vi "RadarAudioPlug+bluetooth.vi"() -> ()   [LabVIEW 2012]
doc: "This VI illustrates how to acquire sound samples continuously from a specified device. It requires the use of a microphone attached to the sound card. You can specify the number of samples to acquire, sample rate, number of channels and a bit rate per sample. The VI also plots the raw data as the acquisition is made."
uses:
  <vilib>/sound2/lvsound2.llb/Sound Data Format.ctl
  <vilib>/Analysis/4window.llb/windowTd.ctl
  <vilib>/sound2/lvsound2.llb/Sampling Mode.ctl
  <vilib>/Instr/_visa.llb/VISA Configure Serial Port (Instr).vi
  <vilib>/sound2/lvsound2.llb/Sound Input Read (DBL).vi
  <vilib>/gmath/NI_Gmath.lvlib
  <vilib>/ptbypt/NI_PtbyPt.lvlib
  <vilib>/Analysis/NI_AALPro.lvlib
panel:
  in  "Enable Termination\nChar (T)":bool=TRUE
  out "read buffer":string
  out "I/Q signal":dynamicdata(graph)
  in  "?":bool
  in  "flow control":u16(ring) items=["None"=0, "XON/XOFF"=1, "RTS/CTS"=2, "DTR/DSR"=4]
  in  "Input\nbuffer size":u32=4096
  in  "termination char\n(0xA = '\\n' = LF)":u8=10 format="%.0x"
  in  "timeout (ms)":u32=10000
  in  "stop bits":u16(ring)=10 items=["1.0"=10, "1.5"=15, "2.0"=20]
  in  "parity":u16(ring) items=["None", "Odd", "Even", "Mark", "Space"]
  in  "data bits":u16=8 min=5 max=8 step=1
  in  "VISA resource name":refnum<visa-resource-name>="COM1"
  in  "baud rate":u32=115200
  in  "start time":timestamp
  in  "stop time":timestamp
  out "STFT Spectrogram":dbl[][](graph)
  in  "Save data":bool=TRUE caption="Enable"
  in  "window info":cluster{"type":T1, "length":i32}={"type"=1, "length"=64} {"type" items=["Rectangle"=0, "Hanning"=1, "Hamming"=2, "Blackman-Harris"=3, "Exact Blackman"=4, "Blackman"=5, "Flat Top"=6, "4 Term B-Harris "=7, "7 Term B-Harris"=8, "Low Sidelobe"=9, "Blackman Nuttall"=11, "Triangle"=30, "Bartlett-Hanning"=31, "Bohman"=32, "Parzen"=33, "Welch"=34, "Kaiser"=60, "Dolph-Chebyshev"=61, "Gaussian"=62]}
  in  "time-freq sampling info":cluster{"time steps":i32, "frequency bins":i32}={"time steps"=-1, "frequency bins"=512}
  in  "Sound Format":T2={"sample rate (S/s)"=22050.0, "number of channels"=2, "bits per sample"=16}
  out "Raw Data":waveform(dbl)[](graph)
  in  "stop":bool
  in  "Device ID":u32 format="%.0x"
  in  "Number of Samples/ch":i32=5000
  # "Configuration"
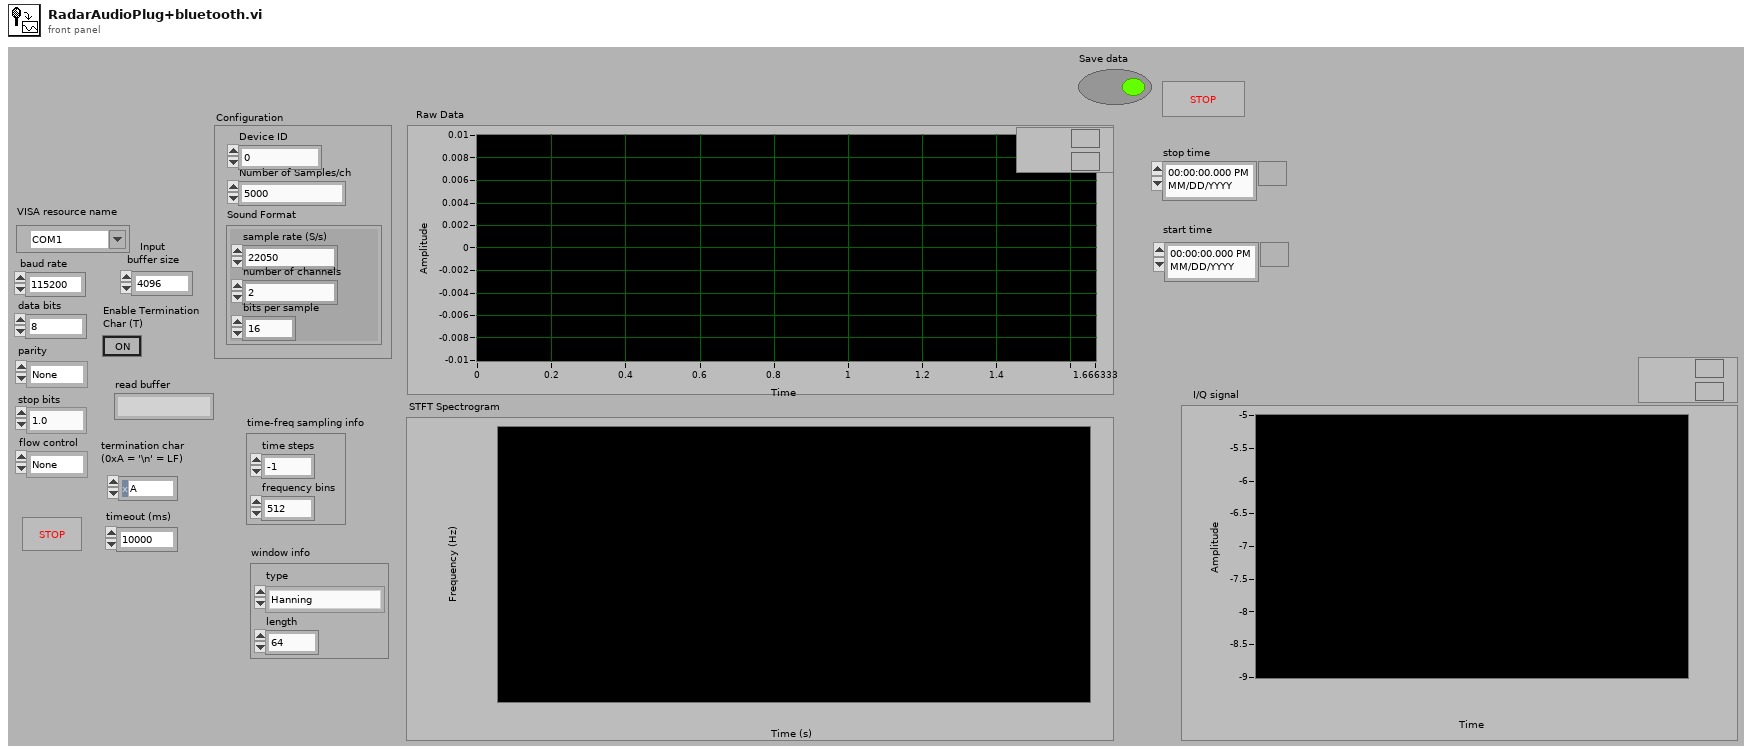
[diagram p1: front panel]
types:
  T1 = typedef "NI_AALPro.lvlib/windowTd.ctl" = u32
  T2 = typedef "Sound Data Format.ctl" = cluster{"sample rate (S/s)":dbl, "number of channels":i32, "bits per sample":i32}
  T3 = typedef "Sampling Mode.ctl" = i32
  T4 = typedef "Sound Input Task ID.ctl" = u32
  T5 = enum16{"fire", "rainbow", "grey", "inverse grey", "ice", "original"}
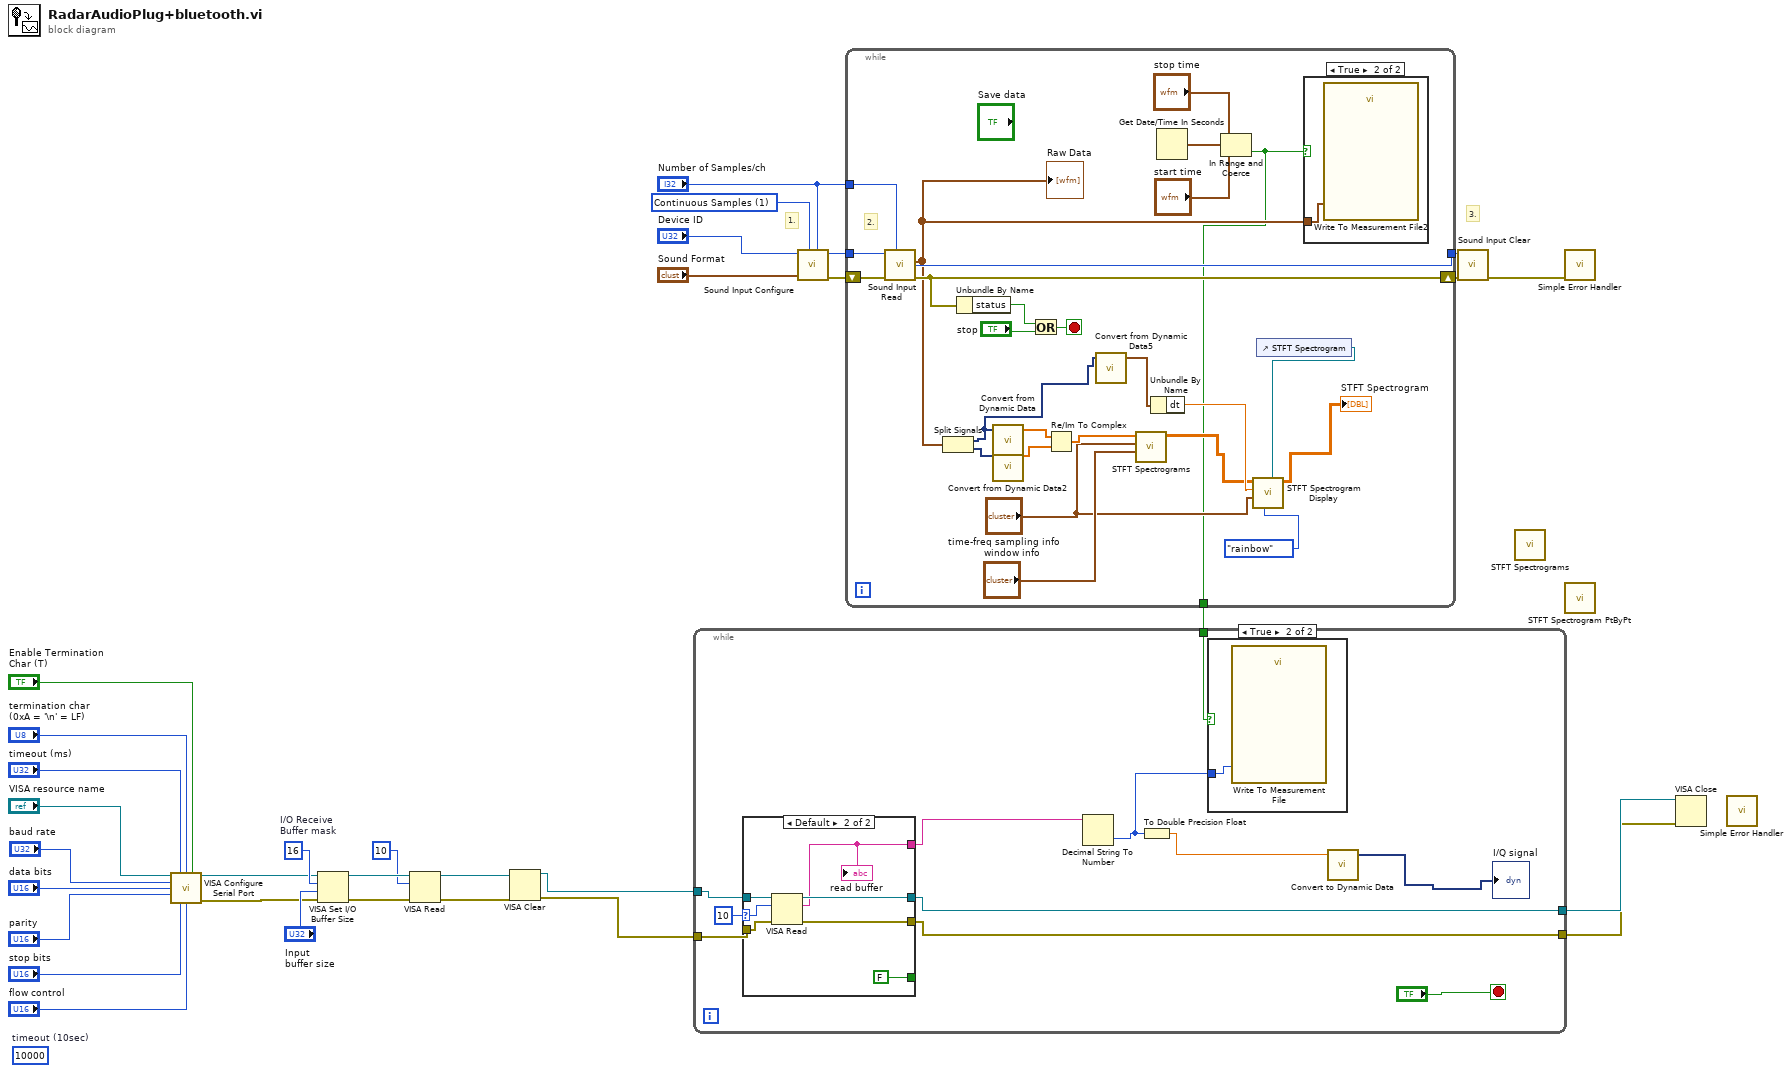
[diagram p0: block diagram]
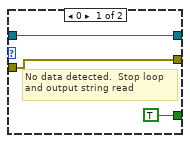
[diagram p3: hidden frame]
diagram:
  (unwired) u32 10000  # timeout (10sec)
  w18 = u16 16  # I/O Receive Buffer mask
  w27 = T3 1 items=["Finite Samples", "Continuous Samples"] ("sample mode")
  # "3."
  # "1."
  n1 = call-poly "VISA Configure Serial Port"("VISA resource name"="VISA resource name", "timeout (10sec)"="timeout (ms)", "termination char\n(0xA = '\\n' = LF)"="termination char\n(0xA = '\\n' = LF)", "Enable Termination\nChar (T)"="Enable Termination\nChar (T)", "baud rate (9600)"="baud rate", "data bits (8)"="data bits", "parity (0:none)"="parity", "stop bits (10: 1 bit)"="stop bits", "flow control (0:none)"="flow control") -> ("VISA resource name out"=w13:refnum<visa-resource-name>, "error out"=w12:errorcluster)  [unwired: 1 in, 4 out]
  n2 = VISA Set I/O Buffer Size(VISA resource name=w13, mask (16)=w18, size (4096)="Input\nbuffer size", error in (no error)=w12) -> (VISA resource name out=w11:refnum<visa-resource-name>, error out=w10:errorcluster)
  n3 = VISA Read(VISA resource name=w11, byte count=u32 10, error in (no error)=w10) -> (VISA resource name out=w7:refnum<visa-resource-name>, error out=w6:errorcluster)  [unwired: 2 out]
  n4 = VISA Clear(VISA resource name=w7, error in (no error)=w6) -> (VISA resource name out=w5:refnum<visa-resource-name>, error out=w4:errorcluster)
  n5 = call <vilib>:"Sound Input Configure.vi"("number of samples/ch"="Number of Samples/ch", "sample mode"=w27, "sound format"="Sound Format", "device ID"="Device ID") -> ("error out"=w32:errorcluster, "task ID"=w30:T4)  [unwired: 3 in, 3 out]
  n6 = while {
    tunnel: w30 -> [w57]
    tunnel: [w56] -> w29
    tunnel: "Number of Samples/ch" -> [w55]
    shift-right: [w51] -> w28
    shift-left: w32 -> [w58]
    tunnel: [w33] -> w1
    stop <- w52 stop-if-true
    # "2."
    n7 = call-poly <vilib>:"Sound Input Read.vi"("number of samples/ch"=w55, "error in (no error)"=w58, "task ID"=w57) -> ("error out"=w51:errorcluster, "data"=w34:waveform(dbl)[], "task ID out"=w56:T4)  [unwired: 1 in, 5 out]
    "Raw Data" <- w34
    n8 = Split Signals(w34) -> (w45:dynamicdata, w46:dynamicdata)  [unwired: 2 out]
    n9 = Unbundle By Name(w51) -> ("status"=w54:bool)
    n10 = call "Convert from Dynamic Data"("Dynamic Data Type"=w45) -> ("Array"=w47:dbl[])  [unwired: 3 out]
    n11 = call "Convert from Dynamic Data2"("Dynamic Data Type"=w46) -> ("Array"=w50:dbl[])  [unwired: 3 out]
    n12 = Or(x=w54, y="stop") -> (x .or. y?=w52:bool)
    n13 = Re/Im To Complex(1:w50, 2:w47) -> (0:w49:cdb[])
    n14 = call "Convert from Dynamic Data5"("Dynamic Data Type"=w45) -> ("Waveform"=w44:waveform(dbl))  [unwired: 1 in, 2 out]
    n15 = call <vilib>:"STFT Spectrograms.vi"("window info"="window info", "time-freq sampling info"="time-freq sampling info", "X"=w49) -> ("STFT Spectrogram {X}"=w42:dbl[][])  [unwired: 3 in, 5 out]
    n16 = Unbundle By Name(w44) -> ("dt"=w43:dbl)
    n17 = Get Date/Time In Seconds() -> (seconds since 1Jan1904=w37:timestamp)
    n18 = In Range and Coerce(upper limit="stop time", x=w37, lower limit="start time") -> (In Range?=w33:bool)  [unwired: 1 out]
    n19 = control-ref of="STFT Spectrogram"() -> (w39:refnum<vi>)
    n20 = call "STFT Spectrogram Display.vi"("Intensity Graph"=w39, "map selector"=T5."rainbow", "time-freq sampling info"="time-freq sampling info", "dt"=w43, "STFT Spectrogram In"=w42) -> ("STFT Spectrogram Out"=→"STFT Spectrogram":dbl[][])  [unwired: 2 in, 4 out]
    n21 = case shown="True" w33 {
      tunnel: w34 -> [_ w59]
      frame False {
      }
      frame True {
        n22 = call "Write To Measurement File2"("Signals"=w59) -> ()  [unwired: 16 in, 3 out]
      }
    }
  }
  n23 = while {
    tunnel: w5 -> [w70]
    tunnel: w4 -> [w69]
    tunnel: [w64] -> w3
    tunnel: [w63] -> w2
    tunnel: w1 -> [w60]
    stop <- "?" stop-if-true
    n24 = case shown="Default" u32 10 ("Bytes at Port") {
      selector: u32 10 ("Bytes at Port") -> [_ w77]
      tunnel: [TRUE FALSE] -> _
      tunnel: [w72 w80] -> w63
      tunnel: [w73 w79] -> w64
      tunnel: [_ w78] -> w66
      tunnel: w70 -> [w73 w76]
      tunnel: w69 -> [w72 w75]
      frame 0 {
        # "No data detected.  Stop loop\nand output string read"
      }
      frame Default {
        n25 = VISA Read(VISA resource name=w76, byte count=w77, error in (no error)=w75) -> (VISA resource name out=w79:refnum<visa-resource-name>, read buffer=w78:string, error out=w80:errorcluster)  [unwired: 1 out]
        "read buffer" <- w78
      }
    }
    n26 = Decimal String To Number(string=w66) -> (number=w61:i32)  [unwired: 1 in, 2 out]
    n27 = To Double Precision Float(number=w61) -> (double precision float=w62:dbl)
    n28 = case shown="True" w60 {
      tunnel: w61 -> [_ w71]
      frame False {
      }
      frame True {
        n29 = call "Write To Measurement File"("Signals"=w71) -> ()  [unwired: 16 in, 3 out]
      }
    }
    n30 = call "Convert to Dynamic Data"("Double"=w62) -> ("Dynamic Data Type"=→"I/Q signal":dynamicdata)  [unwired: 3 in]
  }
  n31 = call <vilib>:"Sound Input Clear.vi"("error in (no error)"=w28, "task ID"=w29) -> ("error out"=w25:errorcluster)  [unwired: 9 out]
  n32 = call <vilib>:"STFT Spectrograms.vi"() -> ()  [unwired: 6 in, 6 out]
  n33 = call <vilib>:"Simple Error Handler.vi"("error in (no error)"=w25) -> ()  [unwired: 1 in, 8 out]
  n34 = call <vilib>:"STFT Spectrogram PtByPt.vi"() -> ()  [unwired: 6 in, 2 out]
  n35 = VISA Close(VISA resource name=w3, error in (no error)=w2) -> ()  [unwired: 1 out]
  n36 = call <vilib>:"Simple Error Handler.vi"() -> ()  [unwired: 2 in, 8 out]
